vi "Get TableName.vi"(8 "error in (no error)":errorcluster, 11 "SQLite_API in":refnum<class "SQLite_API.lvclass">) -> (0 "error out":errorcluster, 2 "TableName List":string[](array[string]), 3 "SQLite_API out":refnum<class "SQLite_API.lvclass">)   [LabVIEW 2021, in "SQLite_API.lvclass"]
uses:
  <userlib>/John_Lib/DataBase/SQLite_API/SQLite_API.lvclass
  <userlib>/John_Lib/DataBase/SQLite_API/SQLite_API.lvclass/SQLite_API.ctl
  <vilib>/drjdpowell/SQLite Library/SQLite.lvlib
  <vilib>/drjdpowell/SQLite Library/SQL Connection/Execute SQL (1D String).vi
  <vilib>/drjdpowell/SQLite Library/SQL Connection/Connection.lvclass
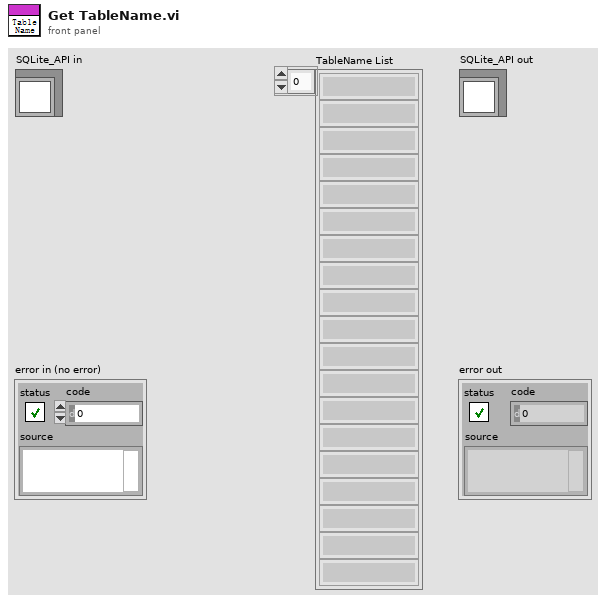
[diagram p1: front panel]
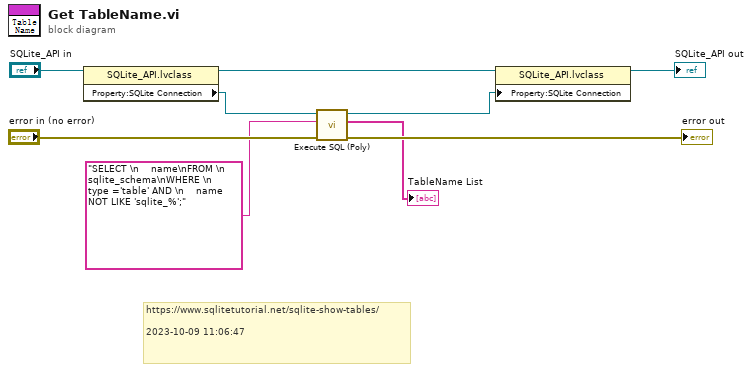
[diagram p0: block diagram]
diagram:
  # "https://www.sqlitetutorial.net/sqlite-show-tables/\n\n2023-10-09 11:06:47"
  n1 = property class="SQLite_API.lvclass"(reference="SQLite_API in") -> (reference out=w8:refnum<class "SQLite_API.lvclass">, "Property:SQLite Connection"=w6:refnum<class "Connection.lvclass">)  [unwired: 1 in, 1 out]
  n2 = call-poly <vilib>:"Execute SQL (Poly).vi"("error in (no error)"="error in (no error)", "SQL"="SELECT \n    name\nFROM \n    sqlite_schema\nWHERE \n    type ='table' AND \n    name NOT LIKE 'sqlite_%';" ("Command Text"), "SQLite Connection in"=w6) -> ("error out"=→"error out":errorcluster, "Result Set"=→"TableName List":string[], "SQLite Connection"=w5:refnum<class "Connection.lvclass">)  [unwired: 5 in, 1 out]
  n3 = property class="SQLite_API.lvclass"(reference=w8, "Property:SQLite Connection"=w5) -> (reference out=→"SQLite_API out":refnum<class "SQLite_API.lvclass">)  [unwired: 1 in, 1 out]
